vi "Free_system.vi"(8 "error in (no error)":errorcluster, 11 "Initialize_card in":refnum<class "Control_card.lvclass">) -> (0 "error out":errorcluster, 3 "Initialize_card out":refnum<class "Control_card.lvclass">)   [LabVIEW 2015, in "Control_card.lvclass"]
uses:
  Control_card.lvclass
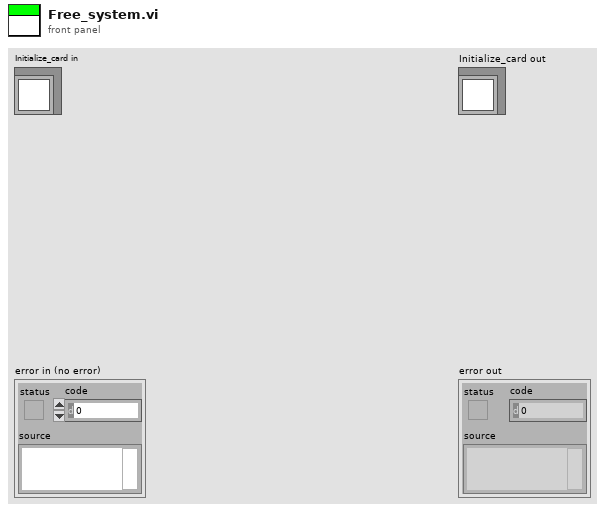
[diagram p1: front panel]
types:
  T1 = cluster{"Handle":u32, "Sample size":u32, "Resolution":i32, "Offset":i32, "Channels":u32, "Boards":u32}
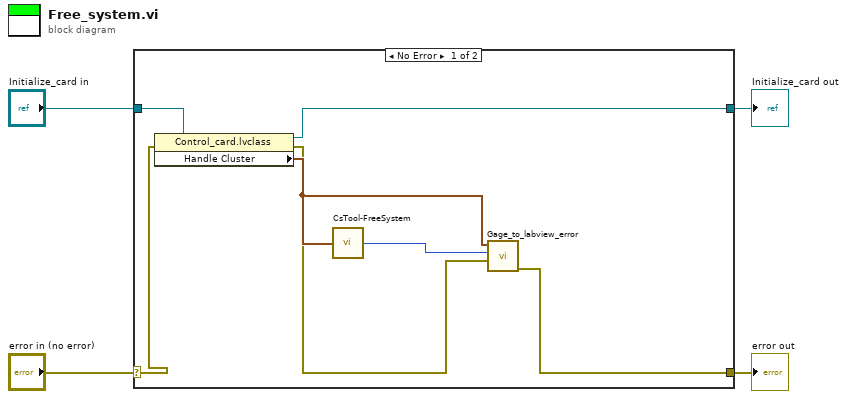
[diagram p0: block diagram]
diagram:
  n1 = case shown="No Error" "error in (no error)" {
    selector: "error in (no error)" -> [w10 w13]
    tunnel: [w5 w13] -> w3
    tunnel: [w9 w12] -> w1
    tunnel: "Initialize_card in" -> [w11 w12]
    frame No Error {
      n2 = property class="Control_card.lvclass"(reference=w11, error in=w10) -> (reference out=w9:refnum<class "Control_card.lvclass">, error out=w6:errorcluster, "Handle Cluster"=w8:T1)
      n3 = call <userlib>:"CsTool-FreeSystem.vi"("Handle Cluster"=w8) -> ("Error Code"=w7:i32)
      n4 = call "Gage_to_labview_error.vi"("Error In"=w6, "GaGe Error Number"=w7, "Handle Cluster"=w8) -> ("Error Out"=w5:errorcluster)  [unwired: 8 in]
    }
    frame Error {
    }
  }
  "error out" <- w3
  "Initialize_card out" <- w1
